vi "E_W_S_N on sphere.vi"(4 "center":cluster{"x":i32, "y":i32}={"x"=51, "y"=51}, 5 "size":i32=40, 7 "rotation":dbl[][](array[numeric]), 9 "pict in":picture) -> (3 "pict out":picture)   [LabVIEW 2011]
uses:
  <vilib>/Analysis/baseanly.llb/Real A x B.vi
  <vilib>/Analysis/NI_AALBase.lvlib
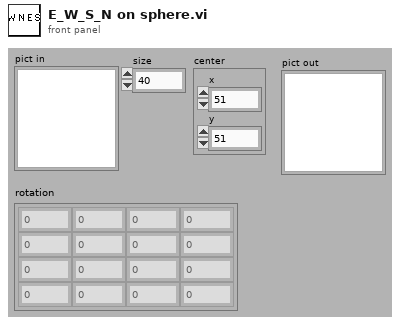
[diagram p1: front panel]
types:
  T1 = cluster{"Width":u16, "Style":enum32{"Solid", "Dash", "Dot", "DashDot", "DashDotDot"}}
  T2 = typedef "NI_Matrix.lvlib/RealMatrix.ctl" = dbl[][]
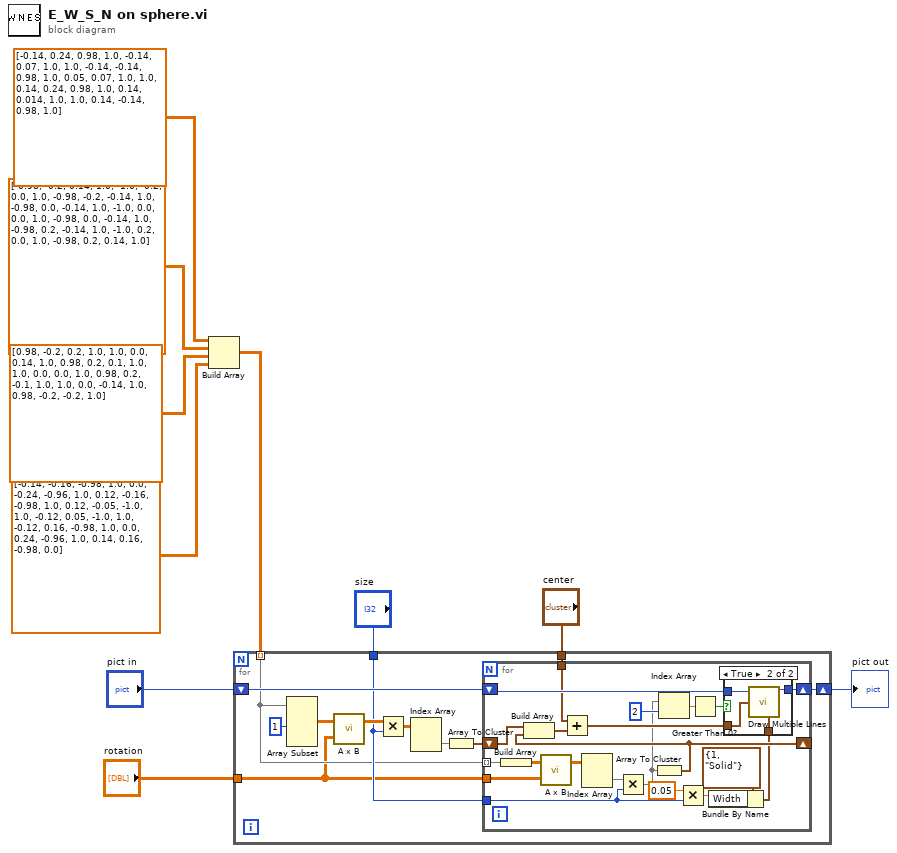
[diagram p0: block diagram]
diagram:
  n1 = Build Array(dbl[][] [[-0.14, 0.24, 0.98, 1.0], [-0.14, 0.07, 1.0, 1.0], [-0.14, -0.14, 0.98, 1.0], [0.05, 0.07, 1.0, 1.0], [0.14, 0.24, 0.98, 1.0], [0.14, 0.014, 1.0, 1.0], [0.14, -0.14, 0.98, 1.0]] ("Array 2"), dbl[][] [[-0.98, -0.2, 0.14, 1.0], [-1.0, -0.2, 0.0, 1.0], [-0.98, -0.2, -0.14, 1.0], [-0.98, 0.0, -0.14, 1.0], [-1.0, 0.0, 0.0, 1.0], [-0.98, 0.0, -0.14, 1.0], [-0.98, 0.2, -0.14, 1.0], [-1.0, 0.2, 0.0, 1.0], [-0.98, 0.2, 0.14, 1.0]] ("Array 2"), dbl[][] [[0.98, -0.2, 0.2, 1.0], [1.0, 0.0, 0.14, 1.0], [0.98, 0.2, 0.1, 1.0], [1.0, 0.0, 0.0, 1.0], [0.98, 0.2, -0.1, 1.0], [1.0, 0.0, -0.14, 1.0], [0.98, -0.2, -0.2, 1.0]] ("Array 2"), dbl[][] [[-0.14, -0.16, -0.98, 1.0], [0.0, -0.24, -0.96, 1.0], [0.12, -0.16, -0.98, 1.0], [0.12, -0.05, -1.0, 1.0], [-0.12, 0.05, -1.0, 1.0], [-0.12, 0.16, -0.98, 1.0], [0.0, 0.24, -0.96, 1.0], [0.14, 0.16, -0.98, 0.0]] ("Array")) -> (w6:dbl[][][])
  n2 = for {
    tunnel: "center" -> [w20]
    tunnel: "size" -> [w16]
    tunnel: w6 -> [w12] mode=indexing
    tunnel: "rotation" -> [w11]
    shift-right: [w21] -> w3
    shift-left: "pict in" -> [w22]
    n3 = Array Subset(array=w12, length (row)=1 ("length")) -> (w14:dbl[][])  [unwired: 3 in]
    n4 = call-poly <vilib>:"A x B.vi"("B"=w11, "A"=w14) -> ("A x B"=w17:T2)  [unwired: 1 out]
    n5 = Multiply(x=w17, y=w16) -> (x*y=w15:T2)
    n6 = Index Array(array=w15) -> (element=w13:dbl[])  [unwired: 2 in]
    n7 = Array To Cluster(array=w13) -> (cluster=w18:cluster{"A x B[0]":dbl, "A x B[1]":dbl})
    n8 = for {
      tunnel: w12 -> [w33] mode=indexing
      tunnel: w11 -> [w34]
      shift-right: [w43] -> _
      shift-left: w18 -> [w42]
      shift-right: [w39] -> w21
      shift-left: w22 -> [w40]
      tunnel: w16 -> [w23]
      tunnel: w20 -> [w38]
      n9 = Build Array(w33) -> (w32:dbl[][])
      n10 = call-poly <vilib>:"A x B.vi"("B"=w34, "A"=w32) -> ("A x B"=w31:T2)  [unwired: 1 out]
      n11 = Index Array(array=w31) -> (element=w30:dbl[])  [unwired: 2 in]
      n12 = Multiply ("Multiply.vi")(x=w30, y=w23) -> (x*y=w29:dbl[])
      n13 = Array To Cluster(array=w29) -> (cluster=w43:cluster{"[0]":dbl, "[1]":dbl})
      n14 = Build Array(w42, w43) -> (w41:cluster{"[0]":dbl, "[1]":dbl}[])
      n15 = Add(x=w38, y=w41) -> (x+y=w37:cluster{dbl, dbl}[])
      n16 = Index Array(array=w29, index=2) -> (element=w35:dbl)
      n17 = Multiply(x=0.05 ("y"), y=w23) -> (x*y=w25:dbl)
      n18 = Greater Than 0?(x=w35) -> (x > 0?=w28:bool)
      n19 = Bundle By Name(cluster=T1 {"Width"=1, "Style"=enum."Solid"} ("pen"), "Width"=w25) -> (w26:T1)
      n20 = case shown="True" w28 {
        tunnel: w40 -> [w44 w48]
        tunnel: [w44 w47] -> w39
        tunnel: w37 -> [_ w46]
        tunnel: w26 -> [_ w45]
        frame False {
        }
        frame True {
          n21 = call <vilib>:"Draw Multiple Lines.vi"("picture"=w48, "line endpoints"=w46, "pen"=w45) -> ("new picture"=w47:picture)  [unwired: 6 in]
        }
      }
    }
  }
  "pict out" <- w3
